vi "手机摄像硬币.vi"() -> ()   [LabVIEW 2018]
uses:
  <vilib>/userdefined/High Color/IMAQdx.ctl
  <vilib>/vision/driver/NI_Vision_Acquisition_Software.lvlib
panel:
  out "Radius":dbl
  in  "相机选择":T1
  out "Image":T2(plugin-control)
  in  "数钱":bool
  out "Money":dbl
  in  "停止":bool
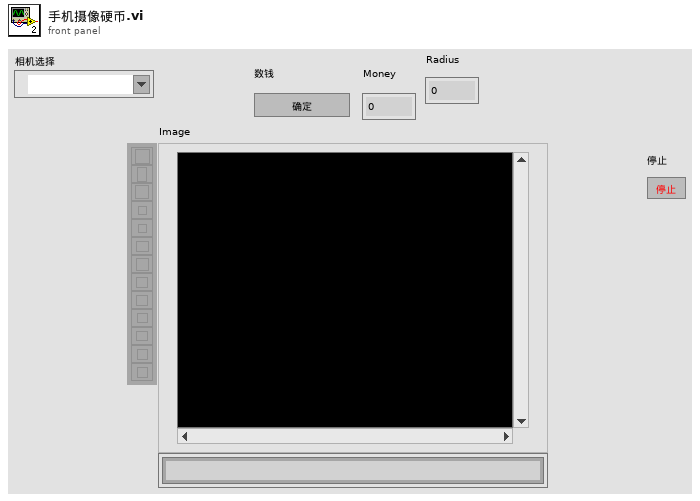
[diagram p1: front panel]
types:
  T1 = typedef "IMAQdx.ctl" = refnum<k21>
  T2 = typedef "IMAQ Image.ctl" = refnum<image>
  T3 = enum16{"Init", "Barcode Input", "Image Processing", "Save Data"}
  T4 = cluster{"Position":cluster{"X":sgl, "Y":sgl}, "Radius":dbl, "Score":dbl}[]
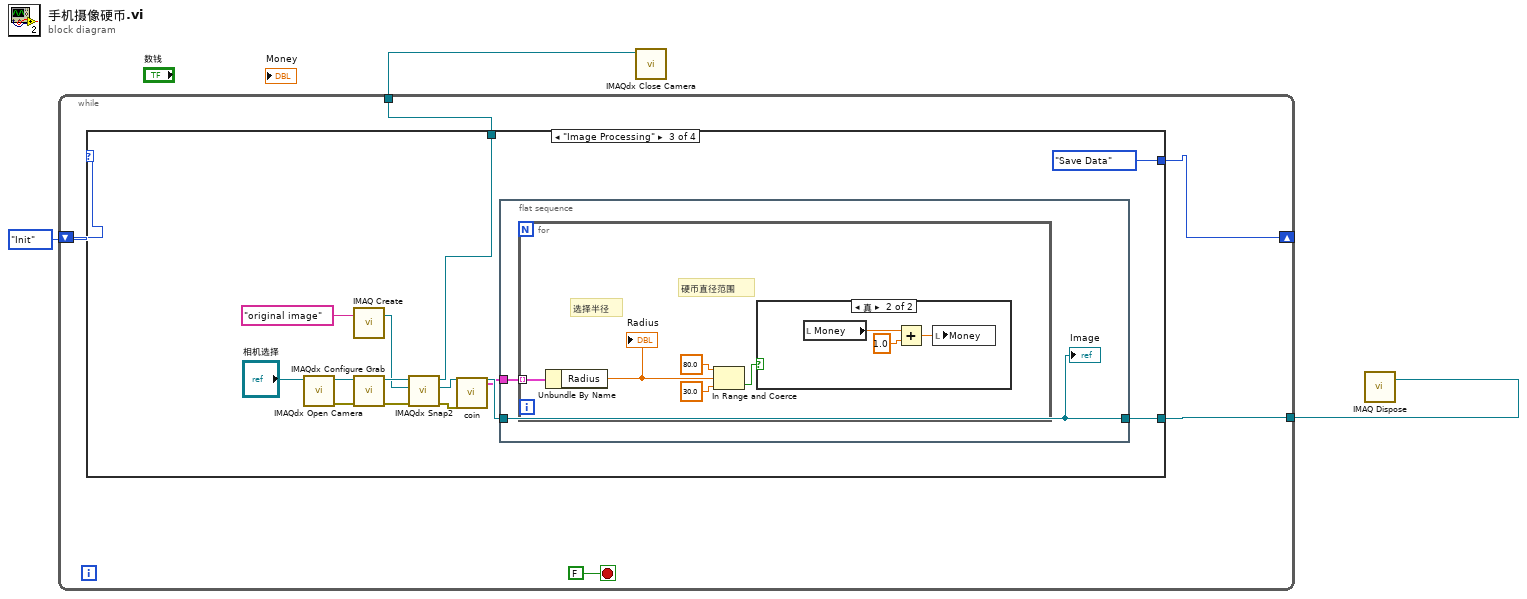
[diagram p0: block diagram]
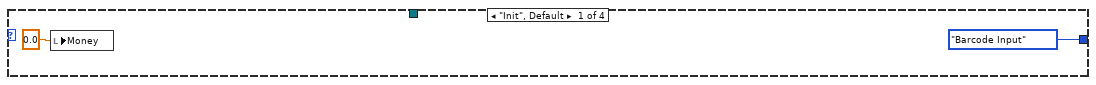
[diagram p2: hidden frame]
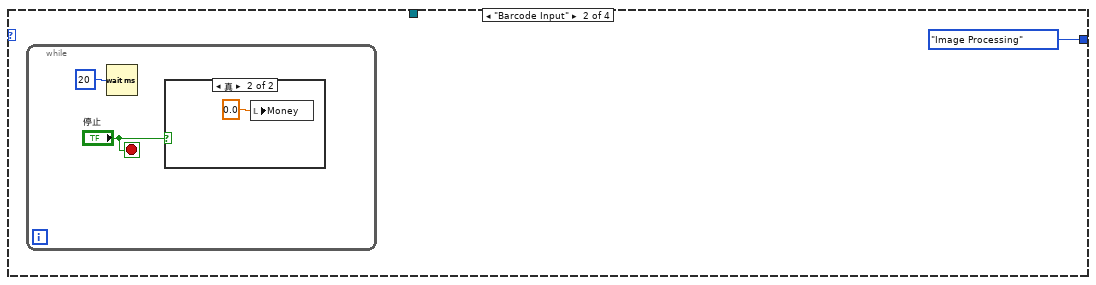
[diagram p3: hidden frame]
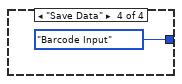
[diagram p6: hidden frame]
diagram:
  n1 = while {
    shift-right: [w6] -> _
    shift-left: T3."Init" ("枚举") -> [w8]
    tunnel: [w5] -> w2
    tunnel: [w4] -> w1
    stop <- FALSE stop-if-true
    n2 = case shown="\"Image Processing\"" w8 {
      tunnel: [T3."Barcode Input" ("枚举") T3."Image Processing" ("枚举") T3."Save Data" ("枚举") T3."Barcode Input" ("枚举")] -> w6
      tunnel: [_ _ w21 _] -> w5
      tunnel: [_ _ w16 _] -> w4
      frame "Init", Default {
        n3 = local write "Money"(0.0 ("Money")) -> ()
      }
      frame "Barcode Input" {
        n4 = while {
          stop <- "停止" stop-if-true
          n5 = Wait (ms)(milliseconds to wait=u32 20 ("等待时间（毫秒）")) -> ()  [unwired: 1 out]
          n6 = case shown="真" "停止" {
            frame False {
            }
            frame True {
              n7 = local write "Money"(0.0 ("Money")) -> ()
            }
          }
        }
      }
      frame "Image Processing" {
        n8 = call <vilib>:"IMAQdx Open Camera.vi"("Session In"="相机选择") -> ("error out"=w25:errorcluster, "Session Out"=w26:T1)  [unwired: 9 in]
        n9 = call "IMAQ Create"("Image Name"="original image") -> ("New Image"=w23:T2)  [unwired: 4 in, 1 out]
        n10 = call <vilib>:"IMAQdx Configure Grab.vi"("error in"=w25, "Session In"=w26) -> ("error out"=w28:errorcluster, "Session Out"=w27:T1)  [unwired: 8 in]
        n11 = call <vilib>:"IMAQdx Snap2.vi"("error in"=w28, "Image In"=w23, "Session In"=w27) -> ("error out"=w18:errorcluster, "Image Out"=w19:T2, "Session Out"=w21:T1)  [unwired: 6 in]
        n12 = call "coin.vi"("Image In"=w19, "error in"=w18) -> ("Image Out"=w17:T2, "Circles (Shape Detection 1)"=w15:T4)  [unwired: 22 in, 2 out]
        n13 = flat-sequence {
          tunnel: w17 -> [w29]
          tunnel: [w29] -> w16
          tunnel: w15 -> [w30]
          frame #0 {
            n14 = for {
              tunnel: w30 -> [w32] mode=indexing
              # "硬币直径范围"
              # "选择半径"
              n15 = Unbundle By Name(w32) -> ("Radius"=w31:dbl)
              "Radius" <- w31
              n16 = In Range and Coerce(upper limit=80.0 ("上限"), x=w31, lower limit=30.0 ("下限")) -> (In Range?=w35:bool)  [unwired: 1 out]
              n17 = case shown="真" w35 {
                frame False {
                }
                frame True {
                  n18 = local read "Money"() -> (w38:dbl)
                  n19 = Add(x=w38, y=1.0) -> (x+y=w36:dbl)
                  n20 = local write "Money"(w36) -> ()
                }
              }
            }
            "Image" <- w29
          }
        }
      }
      frame "Save Data" {
      }
    }
  }
  n21 = call <vilib>:"IMAQdx Close Camera.vi"("Session In"=w2) -> ()  [unwired: 10 in, 1 out]
  n22 = call "IMAQ Dispose"("Image"=w1) -> ()  [unwired: 5 in, 1 out]
